vi "delay.vi"(7 "override":bool, 8 "error in (no error)":errorcluster, 10 "delay (s)":dbl format="%#_16g", 11 "VISA IN":refnum<visa-resource-name>) -> (0 "error out":errorcluster, 2 "value out":dbl=0.000301 format="%#_16p")   [LabVIEW 2017]
uses:
  <instrlib>/Stanford Research DG645/Stanford Research DG645.lvlib
panel:
  in  "channel":u16(ring)=2 items=["A"=2, "B"=3, "C"=4, "D"=5, "E"=6, "F"=7, "G"=8, "H"=9]
  in  "reference":u16(ring) items=["T0"=0, "A"=2, "B"=3, "C"=4, "D"=5, "E"=6, "F"=7, "G"=8, "H"=9]
  in  "VISA (default)":refnum<visa-resource-name>="srs_dg465"
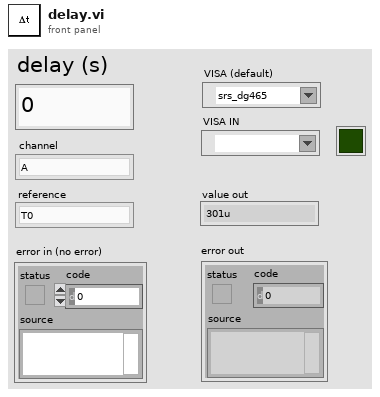
[diagram p1: front panel]
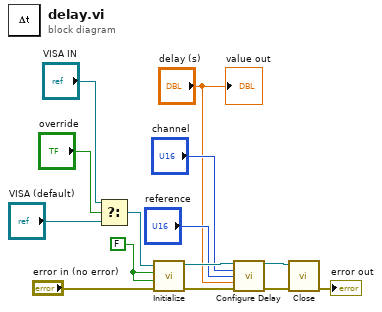
[diagram p0: block diagram]
diagram:
  w8 = FALSE ("Reset (True)")
  n1 = Select(t="VISA IN", s="override", f="VISA (default)") -> (s? t:f=w2:refnum<visa-resource-name>)
  n2 = call <instrlib>:"Initialize.vi"("error in (no error)"="error in (no error)", "Reset (True)"=w8, "ID Query (True)"=w8, "VISA resource name"=w2) -> ("error out"=w12:errorcluster, "VISA resource name out"=w13:refnum<visa-resource-name>)  [unwired: 6 in]
  n3 = call <instrlib>:"Configure Delay.vi"("VISA resource name"=w13, "Channel to Modify (2:A)"="channel", "Reference Channel (0:T0)"="reference", "Delay Time (0 s)"="delay (s)", "error in (no error)"=w12) -> ("VISA resource name out"=w14:refnum<visa-resource-name>, "error out"=w11:errorcluster)  [unwired: 9 in]
  n4 = call <instrlib>:"Close.vi"("error in (no error)"=w11, "VISA resource name"=w14) -> ("error out"=→"error out":errorcluster)  [unwired: 9 in]
  "value out" <- "delay (s)"
